vi "Line Follow.vi"(8 "Initiate":bool, 9 "WristSetpoint":dbl=1500.0 format="%#_13g", 10 "ElevatorSetpoint":dbl=5000.0 format="%#_13g", 11 "ScoreMode in":T1(ring)) -> (3 "element 2":T2)   [LabVIEW 2018]
uses:
  <vilib>/Rock Robotics/WPI/Solenoid/WPI_SolenoidValue.ctl
  <vilib>/Rock Robotics/WPI/Solenoid/WPI_SolenoidSetEnum.vi
  <vilib>/Rock Robotics/WPI/ThirdParty/Phoenix-LabVIEW/Motor Controller/Controls/CTRE_Phoenix_MotorControl_ControlMode.ctl
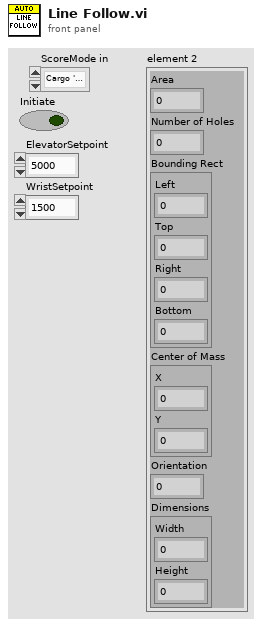
[diagram p1: front panel]
types:
  T1 = enum16{"Cargo 'default'", "Hatch", "HorseDriveHatch"}
  T2 = cluster{"Area":dbl, "Number of Holes":dbl, "Bounding Rect":cluster{"Left":dbl, "Top":dbl, "Right":dbl, "Bottom":dbl}, "Center of Mass":cluster{"X":dbl, "Y":dbl}, "Orientation":dbl, "Dimensions":cluster{"Width":dbl, "Height":dbl}}
  T3 = typedef "WPI_SolenoidValue.ctl" = enum16{"Off", "On", "Forward", "Reverse"}
  T4 = typedef "WPI_CameraDevRef.ctl" = cluster{"Camera Address":string, "CameraStatus":errorcluster}
  T5 = typedef "IMAQ Image.ctl" = refnum<image>
  T6 = typedef "WPI_JoystickDevRef.ctl" = cluster{"Device":T7}
  T7 = typedef "WPI_JoystickDeviceEnum.ctl" = enum16{"USB 0", "USB 1", "USB 2", "USB 3", "USB 4", "USB 5"}
  T8 = typedef "WPI_SolenoidDevRef.ctl" = cluster{"DevStatus":errorcluster, "Pneumatics Control Module":u8, "Forward Solenoid Channel":T9, "Reverse Solenoid Channel":T9}
  T9 = typedef "WPI_SolenoidChannel.ctl" = enum8{"Solenoid 0", "Solenoid 1", "Solenoid 2", "Solenoid 3", "Solenoid 4", "Solenoid 5", "Solenoid 6", "Solenoid 7", "Invalid"}
  T10 = typedef "WPI_MotorControlDeviceRef.ctl" = cluster{"DeviceStatus":errorcluster, "Type":T11, "PWM":cluster{"PWM Channel":T12, "DeadBand":T13}, "CAN":cluster{"Device Number":u8, "SetOutput VI Ref":variant, "GetOutput VI Ref":variant, "Enable VI Ref":variant, "Disable VI Ref":variant, "Data":variant}, "Invert":bool, "DIO PWM":cluster{"PWM \"Enable\" Channel":T12, "DIOChannel":T14, "PWM Rate":dbl}}
  T11 = typedef "WPI_MotorControlType.ctl" = enum16{"PWM", "CAN", "DIO PWM"}
  T12 = typedef "FPGA_DIOPWMChannel.ctl" = enum8{"PWM 0", "PWM 1", "PWM 2", "PWM 3", "PWM 4", "PWM 5", "PWM 6", "PWM 7", "PWM 8", "PWM 9", "PWM MXP 0", "PWM MXP 1", "PWM MXP 2", "PWM MXP 3", "PWM MXP 4", "PWM MXP 5", "PWM MXP 6", "PWM MXP 7", "PWM MXP 8", "PWM MXP 9", "Invalid"}
  T13 = typedef "WPI_PWMDeadband.ctl" = cluster{"Name":string, "maxPositivePwm":i32, "minPositivePwm":i32, "centerPwm":i32, "maxNegativePwm":i32, "minNegativePwm":i32, "angularRange":u16}
  T14 = typedef "FPGA_DIOChannel.ctl" = enum8{"DIO 0", "DIO 1", "DIO 2", "DIO 3", "DIO 4", "DIO 5", "DIO 6", "DIO 7", "DIO 8", "DIO 9", "DIO MXP 0", "DIO MXP 1", "DIO MXP 2", "DIO MXP 3", "DIO MXP 4", "DIO MXP 5", "DIO MXP 6", "DIO MXP 7", "DIO MXP 8", "DIO MXP 9", "DIO MXP 10", "DIO MXP 11", "DIO MXP 12", "DIO MXP 13", "DIO MXP 14", "DIO MXP 15", "SPI Port CS1", "SPI Port CS2", "SPI Port CS3", "SPI Port MISO", "SPI Port MOSI", "Invalid"}
  T15 = typedef "CTRE_Phoenix_MotorControl_ControlMode.ctl" = u16
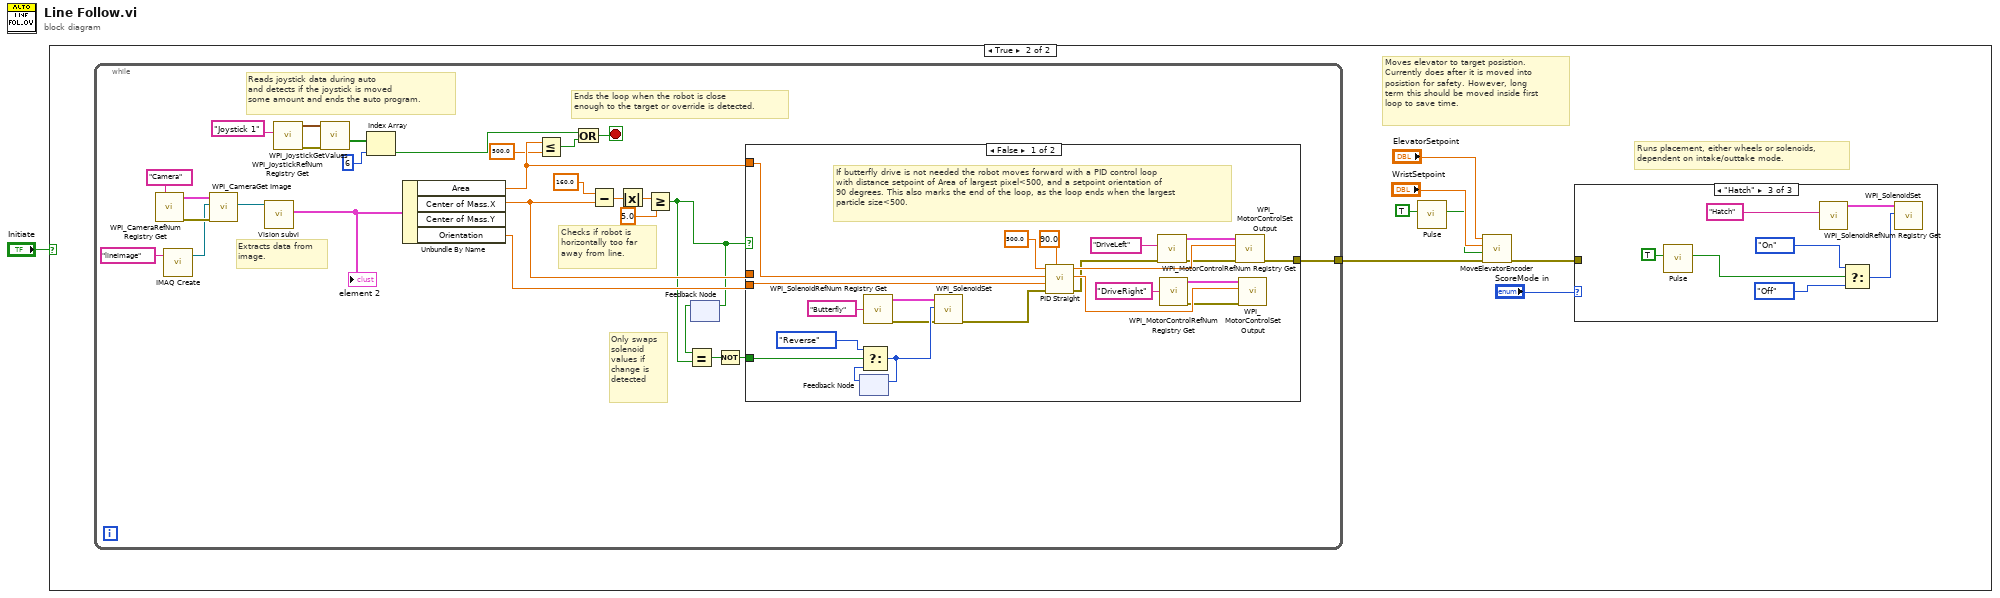
[diagram p0: block diagram]
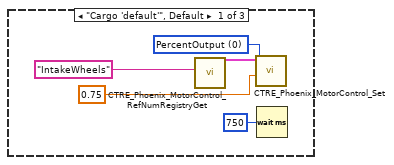
[diagram p3: hidden frame]
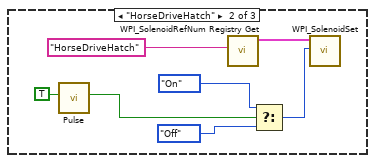
[diagram p4: hidden frame]
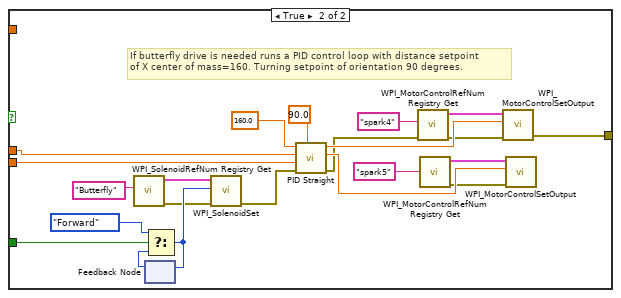
[diagram p5: hidden frame]
diagram:
  n1 = case shown="True" "Initiate" {
    frame False {
    }
    frame True {
      # "Runs placement, either wheels or solenoids,\ndependent on intake/outtake mode."
      # "Moves elevator to target posistion.\nCurrently does after it is moved into\nposistion for safety. However, long\nterm this should be moved inside first\nloop to save time."
      n2 = while {
        tunnel: [w37] -> w3
        stop <- w42 stop-if-true
        # "Only swaps\nsolenoid\nvalues if \nchange is \ndetected"
        # "Checks if robot is \nhorizontally too far \naway from line."
        # "Extracts data from\nimage."
        # "Ends the loop when the robot is close\nenough to the target or override is detected."
        # "Reads joystick data during auto\nand detects if the joystick is moved\nsome amount and ends the auto program."
        n3 = call <vilib>:"WPI_CameraRefNum Registry Get.vi"("refnum name"="Camera") -> ("error out"=w35:errorcluster, "CameraDevRef"=w34:T4)  [unwired: 9 in]
        n4 = call "IMAQ Create"("Image Name"="lineimage") -> ("New Image"=w28:T5)  [unwired: 4 in, 1 out]
        n5 = call <vilib>:"WPI_CameraGet Image.vi"("error in (no error)"=w35, "Image"=w28, "CameraDevRef"=w34) -> ("Image Out"=w36:T5)  [unwired: 6 in, 2 out]
        n6 = call "Vision subvi.vi"("Image Src"=w36) -> ("element 2"=w55:T2)  [unwired: 8 in, 2 out]
        "element 2" <- w55
        n7 = call <vilib>:"WPI_JoystickRefNum Registry Get.vi"("refnum name"="Joystick 1") -> ("error out"=w39:errorcluster, "JoystickDevRef"=w38:T6)  [unwired: 9 in]
        n8 = call <vilib>:"WPI_JoystickGetValues.vi"("error in (no error)"=w39, "JoystickDevRef"=w38) -> ("Buttons"=w32:bool[])  [unwired: 5 in, 4 out]
        n9 = Index Array(array=w32, index=6) -> (element=w31:bool)
        n10 = Unbundle By Name(w55) -> ("Area"=w44:dbl, "Center of Mass.X"=w49:dbl, "Orientation"=w50:dbl)  [unwired: 1 out]
        n11 = Less Or Equal?(x=w44, y=500.0) -> (x <= y?=w41:bool)
        n12 = Or(x=w31, y=w41) -> (x .or. y?=w42:bool)
        n13 = Subtract(x=160.0, y=w49) -> (x-y=w53:dbl)
        n14 = Absolute Value(x=w53) -> (abs(x)=w52:dbl)
        n15 = Greater Or Equal?(x=w52, y=5.0) -> (x >= y?=w47:bool)
        n16 = feedback #1() -> (w48:bool)  [unwired: 1 in]
        n17 = Equal?(x=w48, y=w47) -> (x = y?=w46:bool)
        n18 = feedback-in #1(w47) -> ()
        n19 = Not(x=w46) -> (.not. x?=w45:bool)
        n20 = case shown="False" w47 {
          tunnel: w50 -> [w66 w95]
          tunnel: w49 -> [_ w97]
          tunnel: w44 -> [w65 _]
          tunnel: w45 -> [w63 w84]
          tunnel: [w59 w81] -> w37
          frame False {
            # "If butterfly drive is not needed the robot moves forward with a PID control loop\nwith distance setpoint of Area of largest pixel<500, and a setpoint orientation of\n90 degrees. This also marks the end of the loop, as the loop ends when the largest\nparticle size<500."
            n21 = feedback #2() -> (w61:T3)  [unwired: 1 in]
            n22 = Select(t=WPI_SolenoidValue."Reverse" ("Value"), s=w63, f=w61) -> (s? t:f=w60:T3)
            n23 = feedback-in #2(w60) -> ()
            n24 = call <vilib>:"WPI_SolenoidRefNum Registry Get.vi"("refnum name"="Butterfly") -> ("error out"=w58:errorcluster, "SolenoidDevRef"=w77:T8)  [unwired: 9 in]
            n25 = call-poly <vilib>:"WPI_SolenoidSet.vi"("error in (no error)"=w58, "Value"=w60, "SolenoidDevRef"=w77) -> ("error out"=w76:errorcluster)  [unwired: 7 in, 1 out]
            n26 = call "PID Straight.vi"("Target Angle"=90.0, "Error In"=w76, "Current Angle"=w66, "Current Distance"=w65, "Target Distance"=500.0) -> ("Error Out"=w57:errorcluster, "Right Power"=w68:dbl, "Left Power"=w69:dbl)  [unwired: 4 in]
            n27 = call <vilib>:"WPI_MotorControlRefNum Registry Get.vi"("error in (no error)"=w57, "refnum name"="DriveLeft") -> ("error out"=w56:errorcluster, "MotorControlDevRef"=w70:T10)  [unwired: 8 in]
            n28 = call <vilib>:"WPI_MotorControlRefNum Registry Get.vi"("refnum name"="DriveRight") -> ("error out"=w67:errorcluster, "MotorControlDevRef"=w71:T10)  [unwired: 9 in]
            n29 = call <vilib>:"WPI_MotorControlSetOutput.vi"("error in (no error)"=w56, "Output"=w69, "MotorControlDevRef"=w70) -> ("error out"=w59:errorcluster)  [unwired: 6 in, 2 out]
            n30 = call <vilib>:"WPI_MotorControlSetOutput.vi"("error in (no error)"=w67, "Output"=w68, "MotorControlDevRef"=w71) -> ()  [unwired: 6 in, 3 out]
          }
          frame True {
            # "If butterfly drive is needed runs a PID control loop with distance setpoint\nof X center of mass=160. Turning setpoint of orientation 90 degrees."
            n31 = call <vilib>:"WPI_SolenoidRefNum Registry Get.vi"("refnum name"="Butterfly") -> ("error out"=w80:errorcluster, "SolenoidDevRef"=w99:T8)  [unwired: 9 in]
            n32 = feedback #3() -> (w85:T3)  [unwired: 1 in]
            n33 = Select(t=WPI_SolenoidValue."Forward" ("Value"), s=w84, f=w85) -> (s? t:f=w82:T3)
            n34 = feedback-in #3(w82) -> ()
            n35 = call-poly <vilib>:"WPI_SolenoidSet.vi"("error in (no error)"=w80, "Value"=w82, "SolenoidDevRef"=w99) -> ("error out"=w96:errorcluster)  [unwired: 7 in, 1 out]
            n36 = call "PID Straight.vi"("Target Angle"=90.0, "Error In"=w96, "Current Angle"=w95, "Current Distance"=w97, "Target Distance"=160.0) -> ("Error Out"=w79:errorcluster, "Right Power"=w87:dbl, "Left Power"=w88:dbl)  [unwired: 4 in]
            n37 = call <vilib>:"WPI_MotorControlRefNum Registry Get.vi"("error in (no error)"=w79, "refnum name"="spark4") -> ("error out"=w78:errorcluster, "MotorControlDevRef"=w89:T10)  [unwired: 8 in]
            n38 = call <vilib>:"WPI_MotorControlRefNum Registry Get.vi"("refnum name"="spark5") -> ("error out"=w86:errorcluster, "MotorControlDevRef"=w90:T10)  [unwired: 9 in]
            n39 = call <vilib>:"WPI_MotorControlSetOutput.vi"("error in (no error)"=w78, "Output"=w88, "MotorControlDevRef"=w89) -> ("error out"=w81:errorcluster)  [unwired: 6 in, 2 out]
            n40 = call <vilib>:"WPI_MotorControlSetOutput.vi"("error in (no error)"=w86, "Output"=w87, "MotorControlDevRef"=w90) -> ()  [unwired: 6 in, 3 out]
          }
        }
      }
      n41 = call "Pulse.vi"("Input"=TRUE) -> ("Output"=w4:bool)  [unwired: 10 in]
      n42 = call "MoveElevatorEncoder.vi"("error in (no error)"=w3, 9:w4, "WristSetpoint"="WristSetpoint", "ElevatorSetpoint"="ElevatorSetpoint") -> ("error out"=w2:errorcluster)  [unwired: 7 in]
      n43 = case shown="\"Hatch\"" "ScoreMode in" {
        tunnel: w2 -> [_ _ _]
        frame "Cargo 'default'", Default {
          w11 = T15 0 items=["PercentOutput"=0, "Position"=1, "Velocity"=2, "Current"=3, "Follower"=5, "MotionProfile"=6, "MotionMagic"=7, "MotionProfileArc"=10, "Disabled"=15] ("Control Mode")
          n44 = call <vilib>:"CTRE_Phoenix_MotorControl_RefNumRegistryGet.vi"("refnum name"="IntakeWheels") -> ("PhoenixMotorControlDevRef"=w12:T10)  [unwired: 9 in, 1 out]
          n45 = call <vilib>:"CTRE_Phoenix_MotorControl_Set.vi"("Output"=0.75 ("t"), "Control Mode"=w11, "PhoenixMotorControlDevRef"=w12) -> ()  [unwired: 7 in, 2 out]
          n46 = Wait (ms)(milliseconds to wait=u32 750) -> ()  [unwired: 1 out]
        }
        frame "HorseDriveHatch" {
          n47 = call "Pulse.vi"("Input"=TRUE) -> ("Output"=w15:bool)  [unwired: 10 in]
          n48 = call <vilib>:"WPI_SolenoidRefNum Registry Get.vi"("refnum name"="HorseDriveHatch") -> ("SolenoidDevRef"=w20:T8)  [unwired: 9 in, 1 out]
          n49 = Select(t=WPI_SolenoidValue."On" ("Value"), s=w15, f=WPI_SolenoidValue."Off" ("Value")) -> (s? t:f=w16:T3)
          n50 = call-poly <vilib>:"WPI_SolenoidSet.vi"("Value"=w16, "SolenoidDevRef"=w20) -> ()  [unwired: 8 in, 2 out]
        }
        frame "Hatch" {
          n51 = call "Pulse.vi"("Input"=TRUE) -> ("Output"=w22:bool)  [unwired: 10 in]
          n52 = call <vilib>:"WPI_SolenoidRefNum Registry Get.vi"("refnum name"="Hatch") -> ("SolenoidDevRef"=w27:T8)  [unwired: 9 in, 1 out]
          n53 = Select(t=WPI_SolenoidValue."On" ("Value"), s=w22, f=WPI_SolenoidValue."Off" ("Value")) -> (s? t:f=w23:T3)
          n54 = call-poly <vilib>:"WPI_SolenoidSet.vi"("Value"=w23, "SolenoidDevRef"=w27) -> ()  [unwired: 8 in, 2 out]
        }
      }
    }
  }
